vi "rsp_Msg_ToClient_6.vi"(4 "Show in Debugger?":bool=TRUE, 6 "Message Priority":T1=enum."Normal", 8 "error in":errorcluster, 10 "Data in":T2, 11 "gRPC Client in":refnum<class "gRPC Client.lvclass">) -> (0 "error out":errorcluster, 3 "dup gRPC Client out":refnum<class "gRPC Client.lvclass">)   [LabVIEW 2019, in "gRPC Client (template.proto).lvlib" / "gRPC Client.lvclass"]
doc: "This VI sends a <b>Public API Response</b> message to a registered MHL case of the Caller of the Worker that owns this VI.\n---\nThis Response matches a gRPC message of the same name."
uses:
  gRPC Client.lvclass
  C:/Program Files (x86)/National Instruments/LabVIEW 2019/vi.lib/addons/_Workers/Library/Classes/Worker/Worker.lvclass
  rsp_Msg_ToClient_6.ctl
  Generated_client/RPC Messages/w4lvgrpc_Msg_ToClient_6.ctl
  <vilib>/addons/_Workers/Library/Classes/Message/Priority.ctl
  gRPC Client.lvclass/gRPC Client.ctl
  <vilib>/Utility/error.llb/Error Cluster From Error Code.vi
  <vilib>/addons/_Workers/Library/Classes/Worker/Worker.lvclass
  <vilib>/addons/_Workers/Library/Classes/Message Queue/Message Queue.lvclass
  <vilib>/ErrorRing/Error Ring.xnode
  <vilib>/addons/_Workers/Library/Classes/Message/Message.lvclass
  Generated_client/Generated_client.lvlib
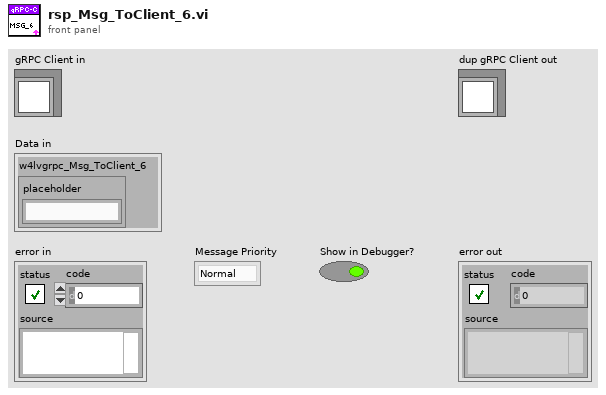
[diagram p1: front panel]
types:
  T1 = typedef "Workers.lvlib/Message.lvclass/Priority.ctl" = enum16{"Low", "Normal", "High"}
  T2 = typedef "gRPC Client (template.proto).lvlib/gRPC Client.lvclass/rsp_Msg_ToClient_6.ctl" = cluster{"w4lvgrpc_Msg_ToClient_6":T3}
  T3 = typedef "Generated_client.lvlib/w4lvgrpc_Msg_ToClient_6.ctl" = cluster{"placeholder":string}
  T4 = typedef "Workers.lvlib/Case Label.ctl" = string
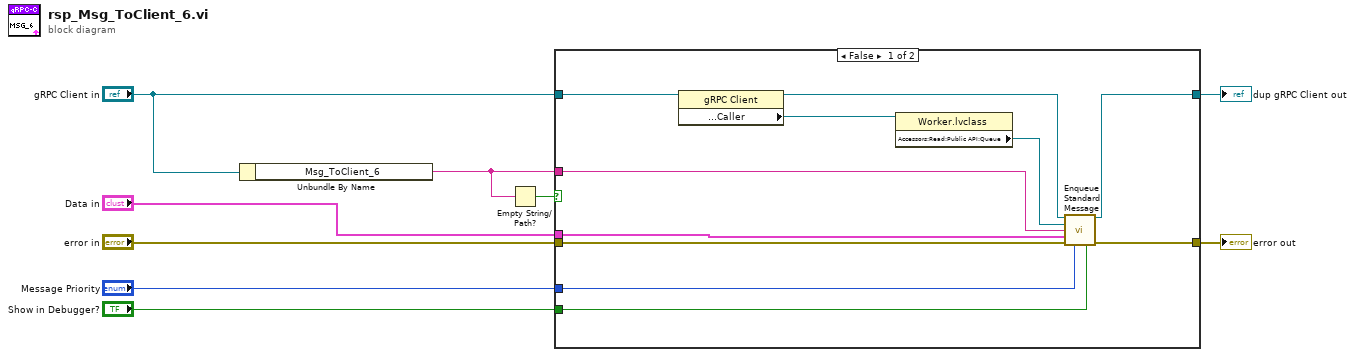
[diagram p0: block diagram]
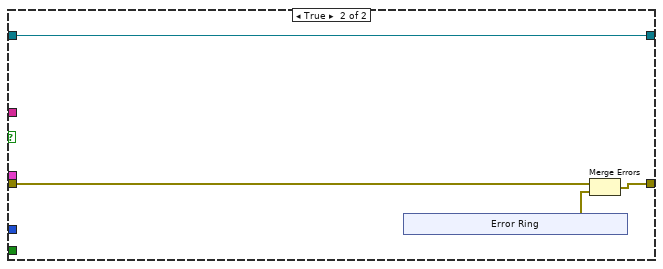
[diagram p2: hidden frame]
diagram:
  n1 = Unbundle By Name("gRPC Client in") -> ("Msg_ToClient_6"=w4:T4)
  n2 = Empty String/Path?(string/path=w4) -> (empty?=w5:bool)
  n3 = case shown="False" w5 {
    tunnel: "error in" -> [w20 w21]
    tunnel: [w19 w22] -> w8
    tunnel: "Data in" -> [w16 _]
    tunnel: [w18 w24] -> w6
    tunnel: "gRPC Client in" -> [w13 w24]
    tunnel: w4 -> [w17 _]
    tunnel: "Show in Debugger?" -> [w15 _]
    tunnel: "Message Priority" -> [w14 _]
    frame False {
      n4 = property class="gRPC Client"(reference=w13) -> (reference out=w12:refnum<class "gRPC Client.lvclass">, "Accessors:Read:Public API:Caller"=w10:refnum<class "Worker.lvclass">)  [unwired: 1 in, 1 out]
      n5 = property class="Worker.lvclass"(reference=w10) -> ("Accessors:Read:Public API:Queue"=w11:refnum<class "Message Queue.lvclass">)  [unwired: 1 in, 2 out]
      n6 = call-dynamic "Enqueue Standard Message.vi"("Worker"=w12, "Message Queue"=w11, "Case Label"=w17, "Data"=w16, "error in (no error)"=w20, "Priority (Normal)"=w14, "Send Message to Debugger? (T)"=w15) -> ("dup Worker out"=w18:refnum<class "gRPC Client.lvclass">, "error out"=w19:errorcluster)  [unwired: 7 in]
    }
    frame True {
      n7 = xnode "Error Ring"() -> ("error out"=w23:errorcluster)
      n8 = Merge Errors(w21, w23) -> (w22:errorcluster)
    }
  }
  "error out" <- w8
  "dup gRPC Client out" <- w6
